vi "Parameter Keys.vi"() -> ()   [LabVIEW 2018, in "Bookmark Manager.lvlib"]
uses:
  Bookmark Manager.lvlib
panel:
  in  "Window Size Key":string="Eulogy.Graveyard.Position"
  in  "Grouping Key":string
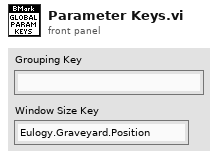
[diagram p1: front panel]
diagram:
